vi "Stage Move Custom Step.vi"(7 "Correlation ID":u32, 8 "error in (no error)":errorcluster, 9 "Axis":T1=enum."Y", 10 "Step (mm)":dbl, 11 "Application in":refnum<class "Application.lvclass">) -> (0 "error out":errorcluster, 3 "Application out":refnum<class "Application.lvclass">)   [LabVIEW 2023, in "Application.lvlib" / "Application.lvclass"]
uses:
  Application.lvclass
  Application.lvclass/Application.ctl
  Hardware/Stage Controller Messages/Move Msg/Move Msg.lvclass
  Hardware/Device Messages/Save CorrID Msg/Save CorrID Msg.lvclass
  Hardware/Stage Controller/Stage Axis.ctl
  Hardware/Stage Controller/Stage Controller.lvclass
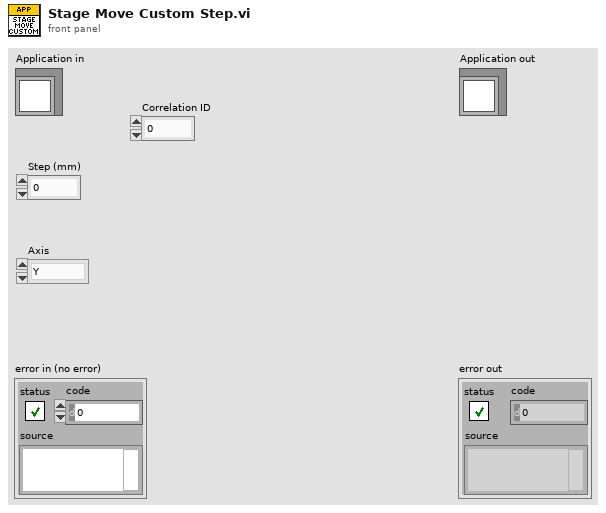
[diagram p1: front panel]
types:
  T1 = typedef "Stage Controller.lvlib/Stage Controller.lvclass/Stage Axis.ctl" = enum16{"unspecified", "X", "Y", "Z"}
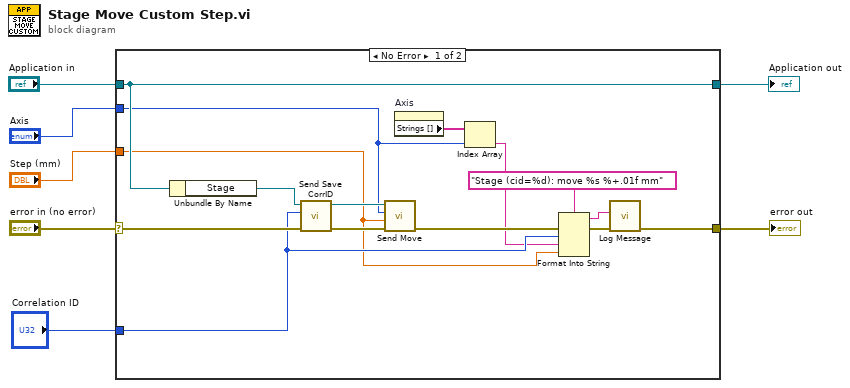
[diagram p0: block diagram]
diagram:
  n1 = case shown="No Error" "error in (no error)" {
    selector: "error in (no error)" -> [w18 w24]
    tunnel: [w13 w24] -> w6
    tunnel: [w22 w23] -> w4
    tunnel: "Application in" -> [w22 w23]
    tunnel: "Step (mm)" -> [w8 _]
    tunnel: "Axis" -> [w10 _]
    tunnel: "Correlation ID" -> [w12 _]
    frame No Error {
      n2 = Unbundle By Name(w22) -> ("Stage"=w19:refnum<class "Message Enqueuer.lvclass">)
      n3 = call "Send Save CorrID.vi"("error in (no error)"=w18, "Correlation ID"=w12, "Message Enqueuer"=w19) -> ("error out"=w21:errorcluster, "Message Enqueuer out"=w20:refnum<class "Message Enqueuer.lvclass">)  [unwired: 7 in]
      n4 = call "Send Move.vi"("error in (no error)"=w21, "Value (mm)"=w8, "Axis"=w10, "Message Enqueuer"=w20) -> ("error out"=w14:errorcluster)  [unwired: 6 in, 1 out]
      n5 = property on="Axis" class="Enum (strict)"() -> ("Strings []"=w11:string[])  [unwired: 2 in, 2 out]
      n6 = Index Array(array=w11, index=w10) -> (element=w9:string)
      n7 = Format Into String(format string="Stage (cid=%d): move %s %+.01f mm", error in=w14, w12, w9, w8) -> (resulting string=w17:string, error out=w15:errorcluster)  [unwired: 1 in]
      n8 = call "Log Message.vi"("error constant"=w15, "input"=w17) -> ("error constant 2"=w13:errorcluster)  [unwired: 8 in, 1 out]
    }
    frame Error {
    }
  }
  "error out" <- w6
  "Application out" <- w4
